vi "Split and Decode JWT.vi"(11 "JWT":string) -> (2 "Payload JSON":string, 3 "Header JSON":string, 5 "Signature":string)   [LabVIEW 2020, in "JWT.lvlib"]
uses:
  JWT.lvlib
  lv-base64/Variant.ctl
  lv-base64/Base64.lvlib
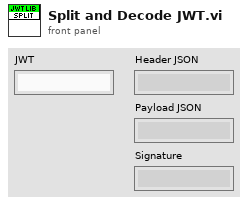
[diagram p1: front panel]
types:
  T1 = typedef "Base64.lvlib/Variant.ctl" = enum16{"Base64", "Base64-URL"}
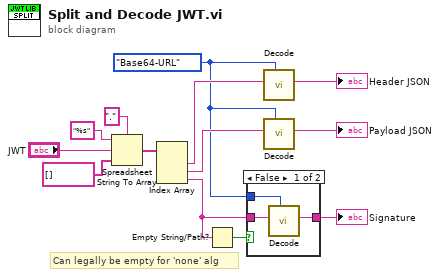
[diagram p0: block diagram]
diagram:
  w8 = Variant."Base64-URL" ("Variant (Base64)")
  # "Can legally be empty for 'none' alg"
  n1 = Spreadsheet String To Array(delimiter (Tab)=".", format string="%s", spreadsheet string="JWT", array type (2D Dbl)=string[] []) -> (array=w11:string[])
  n2 = Index Array(array=w11) -> (element #1=w10:string, element #2=w9:string, element #3=w2:string)  [unwired: 3 in]
  n3 = Empty String/Path?(string/path=w2) -> (empty?=w1:bool)
  n4 = case shown="False" w1 {
    tunnel: w8 -> [w16 _]
    tunnel: w2 -> [w15 w17]
    tunnel: [w14 w17] -> w3
    frame False {
      n5 = call "Decode.vi"("Variant (Base64)"=w16, "string in (base64-encoded)"=w15) -> ("string out (decoded)"=w14:string)  [unwired: 8 in, 1 out]
    }
    frame True {
    }
  }
  "Signature" <- w3
  n6 = call "Decode.vi"("Variant (Base64)"=w8, "string in (base64-encoded)"=w10) -> ("string out (decoded)"=→"Header JSON":string)  [unwired: 8 in, 1 out]
  n7 = call "Decode.vi"("Variant (Base64)"=w8, "string in (base64-encoded)"=w9) -> ("string out (decoded)"=→"Payload JSON":string)  [unwired: 8 in, 1 out]
